vi "ListConfigurationKeys.vi"(8 "error in (no error)":errorcluster, 11 "SMO":refnum<class "SMO.lvclass">) -> (0 "error out":errorcluster, 2 "Keys":string[](array[string]), 3 "SMO out":refnum<class "SMO.lvclass">)   [LabVIEW 2013, in "SMO.lvclass"]
doc: "This method will lookup (and return) the instance reference of <b>Process Name</b>.\n\n---------------------------------------------------------------\nJKI State Machine Objects™\nhttp://jki.net/state-machine-objects/\nCopyright (C) 2005-2015, JKI <info@jki.net>\nALL RIGHTS RESERVED"
uses:
  SMO.lvclass
  Support/Attribute.Config/Attribute.Config.lvclass
panel:
  # "For instructions on how to use the JKI State Machine Objects, examples and video tutorials, visit:\nhttp://jki.net/state-machine-objects/\n\nJKI State Machine Objects™\nhttp://jki.net/state-machine-objects/\nCopyright (C) 2005-2015, JKI <info@jki.net>\nALL RIGHTS RESERVED"
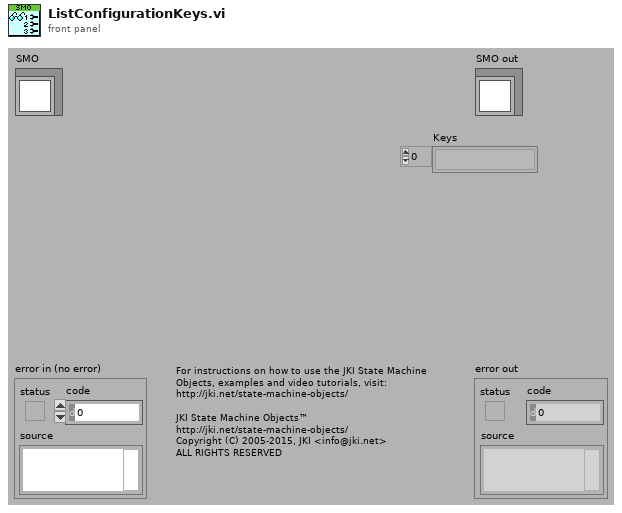
[diagram p1: front panel]
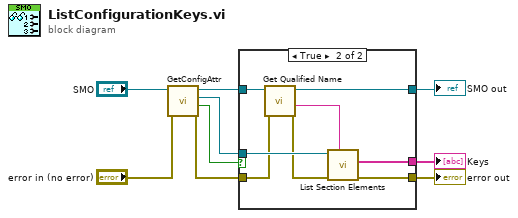
[diagram p0: block diagram]
diagram:
  n1 = call "GetConfigAttr.vi"("error in (no error)"="error in (no error)", "SMO in"="SMO") -> ("error out"=w6:errorcluster, "found"=w8:bool, "Attribute.Config"=w7:refnum<class "Attribute.Config.lvclass">, "SMO out"=w9:refnum<class "SMO.lvclass">)  [unwired: 6 in]
  n2 = case shown="True" w8 {
    tunnel: w7 -> [_ w18]
    tunnel: w9 -> [w11 w16]
    tunnel: [w11 w12] -> w1
    tunnel: w6 -> [w10 w15]
    tunnel: [w10 w19] -> w3
    tunnel: [_ w17] -> w2
    frame False {
    }
    frame True {
      n3 = call "Get Qualified Name.vi"("error in (no error)"=w15, "SMO"=w16) -> ("error out"=w14:errorcluster, "Reserved Qualified Name"=w13:string, "SMO out"=w12:refnum<class "SMO.lvclass">)  [unwired: 6 in, 1 out]
      n4 = call-dynamic "List Section Elements.vi"("Qualified Name"=w13, "error in (no error)"=w14, "Attribute.Config in"=w18) -> ("error out"=w19:errorcluster, "Keys"=w17:string[])  [unwired: 6 in, 1 out]
    }
  }
  "error out" <- w3
  "SMO out" <- w1
  "Keys" <- w2
